vi "ArcadeDriveTeleop.vi"() -> ()   [LabVIEW 2016]
uses:
  <vilib>/Rock Robotics/WPI/Utilities/WPI_GetSetVariantRefNum.vi
  <vilib>/Rock Robotics/WPI/RobotDrive/WPI_RobotDriveArcadeDrive_RatioCurve.vi
panel:
  in  "Sensitivity":dbl=0.5
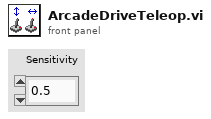
[diagram p1: front panel]
types:
  T1 = typedef "WPI_JoystickDevRef.ctl" = cluster{"Device":T2}
  T2 = typedef "WPI_JoystickDeviceEnum.ctl" = enum16{"USB 0", "USB 1", "USB 2", "USB 3", "USB 4", "USB 5"}
  T3 = typedef "WPI_RobotDriveDevRef.ctl" = cluster{"DevStatus":errorcluster, "Motors[]":T4[], "Square Inputs":bool, "Max Output":dbl}
  T4 = typedef "WPI_MotorControlDeviceRef.ctl" = cluster{"DeviceStatus":errorcluster, "Type":T5, "PWM":cluster{"PWM Channel":T6, "DeadBand":T7}, "CAN":cluster{"Device Number":u8, "SetOutput VI Ref":variant, "GetOutput VI Ref":variant, "Enable VI Ref":variant, "Disable VI Ref":variant, "Data":variant}, "Invert":bool}
  T5 = typedef "WPI_MotorControlType.ctl" = enum16{"PWM", "CAN"}
  T6 = typedef "FPGA_DIOPWMChannel.ctl" = enum8{"PWM 0", "PWM 1", "PWM 2", "PWM 3", "PWM 4", "PWM 5", "PWM 6", "PWM 7", "PWM 8", "PWM 9", "PWM MXP 0", "PWM MXP 1", "PWM MXP 2", "PWM MXP 3", "PWM MXP 4", "PWM MXP 5", "PWM MXP 6", "PWM MXP 7", "PWM MXP 8", "PWM MXP 9", "Invalid"}
  T7 = typedef "WPI_PWMDeadband.ctl" = cluster{"Name":string, "maxPositivePwm":i32, "minPositivePwm":i32, "centerPwm":i32, "maxNegativePwm":i32, "minNegativePwm":i32, "angularRange":u16}
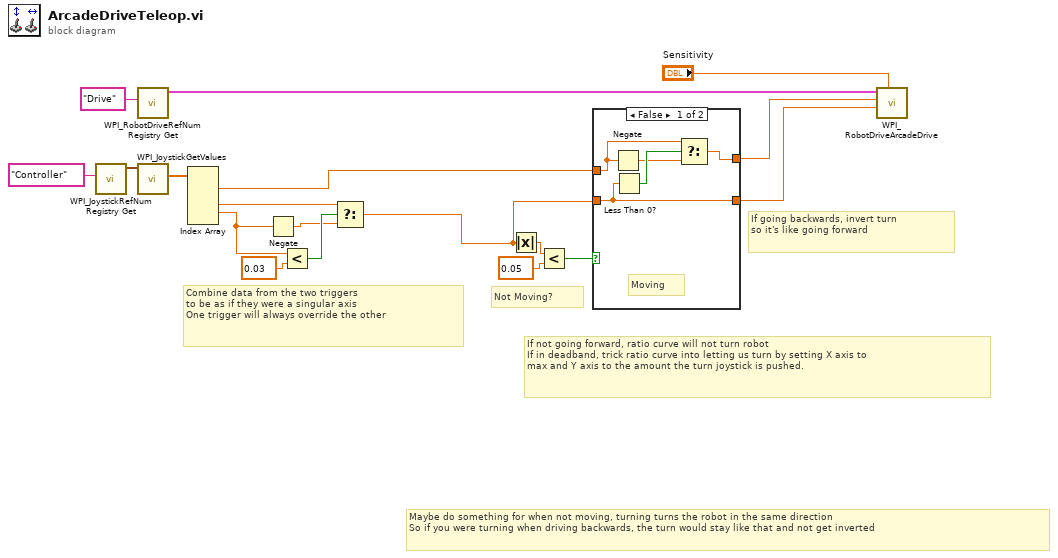
[diagram p0: block diagram]
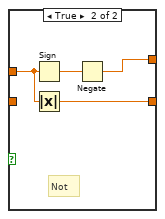
[diagram p2: hidden frame]
diagram:
  # "Maybe do something for when not moving, turning turns the robot in the same direction\nSo if you were turning when driving backwards, the turn would stay like that and not get inverted"
  # "If going backwards, invert turn\nso it's like going forward"
  # "If not going forward, ratio curve will not turn robot\nIf in deadband, trick ratio curve into letting us turn by setting X axis to\nmax and Y axis to the amount the turn joystick is pushed."
  # "Not Moving?"
  # "Combine data from the two triggers\nto be as if they were a singular axis\nOne trigger will always override the other"
  n1 = call <vilib>:"WPI_JoystickRefNum Registry Get.vi"("refnum name"="Controller") -> ("JoystickDevRef"=w12:T1)  [unwired: 9 in, 1 out]
  n2 = call <vilib>:"WPI_RobotDriveRefNum Registry Get.vi"("refnum name"="Drive") -> ("RobotDriveDevRef"=w10:T3)  [unwired: 1 in, 9 out]
  n3 = call <vilib>:"WPI_JoystickGetValues.vi"("JoystickDevRef"=w12) -> ("Axes"=w14:dbl[])  [unwired: 6 in, 4 out]
  n4 = Index Array(array=w14) -> (element #1=w18:dbl, element #3=w7:dbl, element #4=w6:dbl)  [unwired: 5 in, 2 out]
  n5 = Negate(x=w6) -> (-x=w5:dbl)
  n6 = Less?(x=w6, y=0.03) -> (x < y?=w8:bool)
  n7 = Select(t=w7, s=w8, f=w5) -> (s? t:f=w1:dbl)
  n8 = Absolute Value(x=w1) -> (abs(x)=w3:dbl)
  n9 = Less?(x=w3, y=0.05) -> (x < y?=w2:bool)
  n10 = case shown="False" w2 {
    tunnel: [w22 w27] -> w16
    tunnel: [w23 w24] -> w17
    tunnel: w18 -> [w20 w26]
    tunnel: w1 -> [w22 _]
    frame False {
      # "Moving"
      n11 = Negate(x=w20) -> (-x=w19:dbl)
      n12 = Less Than 0?(x=w22) -> (x < 0?=w21:bool)
      n13 = Select(t=w20, s=w21, f=w19) -> (s? t:f=w23:dbl)
    }
    frame True {
      # "Not"
      n14 = Sign(1:w26) -> (0:w25:dbl)
      n15 = Absolute Value(x=w26) -> (abs(x)=w27:dbl)
      n16 = Negate(x=w25) -> (-x=w24:dbl)
    }
  }
  n17 = call-poly <vilib>:"WPI_RobotDriveArcadeDrive.vi"("Sensitivity"="Sensitivity", "Y axis value (Speed)"=w16, "X axis value (Curve)"=w17, "RobotDriveDevRef"=w10) -> ()  [unwired: 5 in, 3 out]
